vi "2L09-OBS_N(t).vi"(10 "dN":dbl[](array[numeric]), 11 "t":dbl[](array[numeric])) -> (2 "N(t)":dbl[](array[numeric]), 3 "t":dbl[](array[numeric]))   [LabVIEW 2010, in "lv_02.lvlib"]
uses:
  lv_02.lvlib
  lv_01/lv_01.lvlib
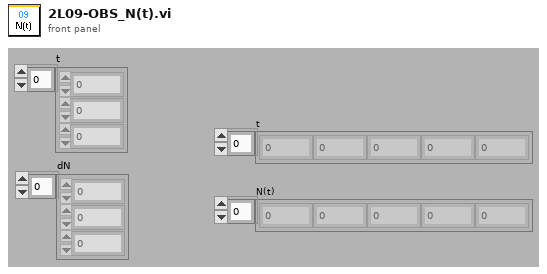
[diagram p1: front panel]
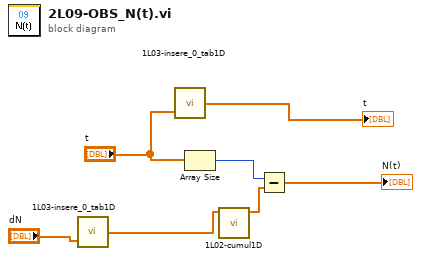
[diagram p0: block diagram]
diagram:
  n1 = call "1L03-insere_0_tab1D.vi"("t"="dN") -> ("t"=w6:dbl[])  [unwired: 1 in]
  n2 = call "1L03-insere_0_tab1D.vi"("t"="t") -> ("t"=→"t":dbl[])  [unwired: 1 in]
  n3 = Array Size(array="t") -> (size(s)=w3:i32)
  n4 = call "1L02-cumul1D.vi"("X"=w6) -> ("X Cum"=w7:dbl[])  [unwired: 3 in, 3 out]
  n5 = Subtract(x=w3, y=w7) -> (x-y=→"N(t)":dbl[])
